vi "Global_var.vi"() -> ()   [LabVIEW 2014]
uses:
  ctl/Point.ctl
  ctl/P3AT_Current.ctl
  ctl/Global_Goal.ctl
panel:
  in  "模拟":bool
  in  "Ini_maxvel":dbl
  in  "address":string="192.168.1.117"
  in  "Global_Planner_Recyle":dbl
  in  "P3AT_Current_Pose":T1
  in  "Last_Global_Goal":T2
  in  "Global_Goal":T2
  in  "P3AT_Current":T3={"max_vel"=0.49056603773584906, "max_rot"=0.5094339622641509, "now_pose_X"=0.0, "now_pose_Y"=0.0, "now_pose_Rot_deg"=0.0, "Control_Mode"=enum."Undefined"} {"max_rot" scale=0.0..1.0; "max_vel" scale=0.0..1.0}
  in  "Last_Local_Goal":T4
  in  "Local_Goal":T4
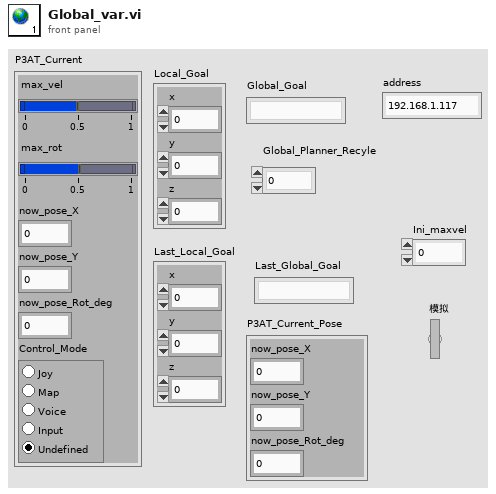
[diagram p1: front panel]
types:
  T1 = cluster{"now_pose_X":dbl, "now_pose_Y":dbl, "now_pose_Rot_deg":dbl}
  T2 = typedef "Global_Goal.ctl" = string
  T3 = typedef "P3AT_Current.ctl" = cluster{"max_vel":dbl, "max_rot":dbl, "now_pose_X":dbl, "now_pose_Y":dbl, "now_pose_Rot_deg":dbl, "Control_Mode":enum32{"Joy", "Map", "Voice", "Input", "Undefined"}}
  T4 = typedef "Point.ctl" = cluster{"x":dbl, "y":dbl, "z":dbl}
diagram:
